vi "LJstreamUD build header string.vi"(8 "Disable Scaling":bool=TRUE, 11 "Channel Config":T1={"# Channels"=4, "+Ch"=["0", "1", "2", "3", "4", "5", "6", "7"], "-Ch (U3)"=["31", "31", "31", "31", "31", "31", "31", "31"], "Ranges (UE9)"=[0, 0, 0, 0, 0, 0, 0, 0], "Scaling Equation"=["y=v0", "y=v1", "y=v2", "y=v3", "y=v4", "y=v5", "y=v6", "y=v7"]} {"Ranges (UE9)" items=["LJ_rgBIP5V", "LJ_rgUNI5V", "LJ_rgUNI2P5V", "LJ_rgUNI1P25V", "LJ_rgUNIP625V"]}) -> (3 "Header String":string)   [LabVIEW 2020]
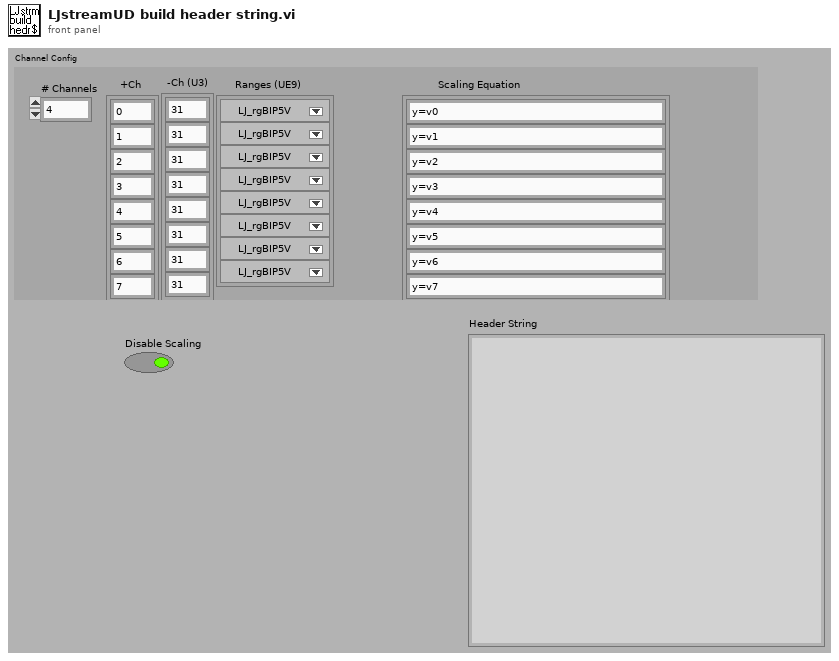
[diagram p1: front panel]
types:
  T1 = cluster{"# Channels":i32, "+Ch":string[], "-Ch (U3)":string[], "Ranges (UE9)":u16[], "Scaling Equation":string[]}
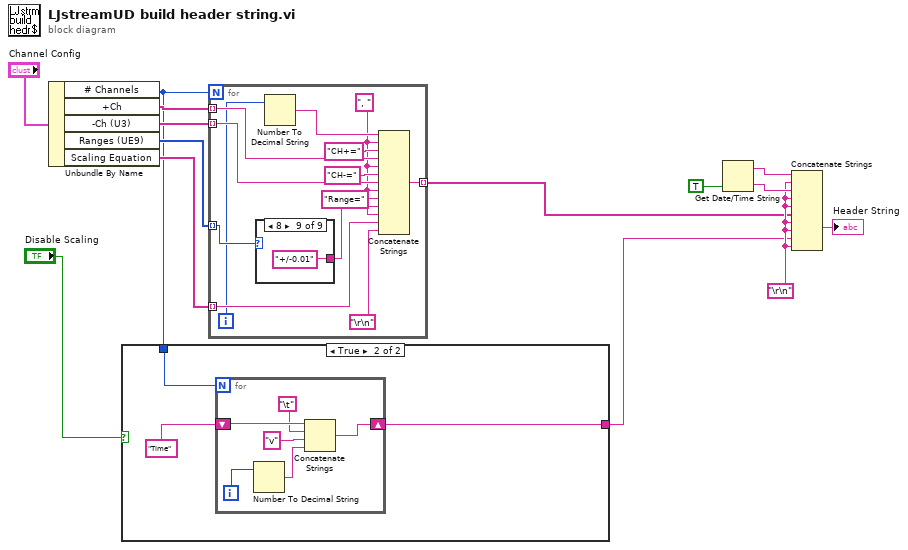
[diagram p0: block diagram]
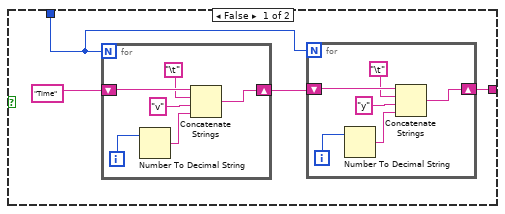
[diagram p2: hidden frame]
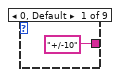
[diagram p3: hidden frame]
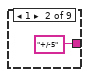
[diagram p4: hidden frame]
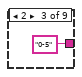
[diagram p5: hidden frame]
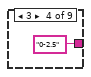
[diagram p6: hidden frame]
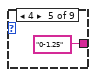
[diagram p7: hidden frame]
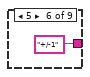
[diagram p8: hidden frame]
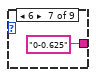
[diagram p9: hidden frame]
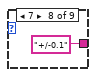
[diagram p10: hidden frame]
diagram:
  w12 = "\r\n"
  n1 = Unbundle By Name("Channel Config") -> ("# Channels"=w5:i32, "+Ch"=w9:string[], "-Ch (U3)"=w8:string[], "Ranges (UE9)"=w6:u16[], "Scaling Equation"=w7:string[])
  n2 = case shown="True" "Disable Scaling" {
    tunnel: w5 -> [w17 w32]
    tunnel: [w15 w31] -> w3
    frame False {
      n3 = for {
        N: w17 -> [_]
        shift-right: [w29] -> w16
        shift-left: "Time" ("Substring") -> [w30]
        i -> [w26]
        n4 = Number To Decimal String(number=w26) -> (decimal integer string=w25:string)  [unwired: 1 in]
        n5 = Concatenate Strings(w30, "\t", "v" ("Substring"), w25) -> (w29:string)
      }
      n6 = for {
        N: w17 -> [_]
        shift-right: [w23] -> w15
        shift-left: w16 -> [w24]
        i -> [w20]
        n7 = Number To Decimal String(number=w20) -> (decimal integer string=w19:string)  [unwired: 1 in]
        n8 = Concatenate Strings(w24, "\t", "y" ("Substring"), w19) -> (w23:string)
      }
    }
    frame True {
      n9 = for {
        N: w32 -> [_]
        shift-right: [w38] -> w31
        shift-left: "Time" ("Substring") -> [w39]
        i -> [w35]
        n10 = Number To Decimal String(number=w35) -> (decimal integer string=w34:string)  [unwired: 1 in]
        n11 = Concatenate Strings(w39, "\t", "v" ("Substring"), w34) -> (w38:string)
      }
    }
  }
  n12 = for {
    N: w5 -> [_]
    tunnel: w9 -> [w50] mode=indexing
    tunnel: w8 -> [w48] mode=indexing
    tunnel: w7 -> [w46] mode=indexing
    tunnel: w6 -> [w45] mode=indexing
    tunnel: [w41] -> w4 mode=indexing
    i -> [w40]
    w47 = ", " ("Substring")
    n13 = case shown="8" w45 {
      tunnel: ["+/-10" "+/-5" "0-5" "0-2.5" "0-1.25" "+/-1" "0-0.625" "+/-0.1" "+/-0.01"] -> w43
      frame 0, Default {
      }
      frame 1 {
      }
      frame 2 {
      }
      frame 3 {
      }
      frame 4 {
      }
      frame 5 {
      }
      frame 6 {
      }
      frame 7 {
      }
      frame 8 {
      }
    }
    n14 = Number To Decimal String(number=w40) -> (decimal integer string=w52:string)  [unwired: 1 in]
    n15 = Concatenate Strings(w52, w47, "CH+=" ("Substring"), w50, w47, "CH-=" ("Substring"), w48, w47, "Range=" ("Substring"), w43, w47, w46, "\r\n") -> (w41:string)
  }
  n16 = Get Date/Time String(want seconds? (F)=TRUE) -> (date string=w14:string, time string=w13:string)  [unwired: 2 in]
  n17 = Concatenate Strings(w14, w12, w13, w12, w12, w4, w12, w12, w3, w12) -> (→"Header String":string)
